vi "Create Dis.vi"(0 "reference in":refnum<class "Stand.lvclass">, 11 "error in (no error)":errorcluster) -> (4 "reference out":refnum<class "Stand.lvclass">, 15 "error out":errorcluster)   [LabVIEW 2019, in "Stand.lvclass"]
uses:
  Stand.lvclass
  C:/Users/ANENKOV_V1/Desktop/src/Proccess_class/Proccess.lvclass
  Stand.lvclass/Stand.ctl
  Proccess_class/Proccess.lvclass/Proccess.ctl
  Proccess_class/TAGs.ctl
  DI_class/DI.lvclass
  Proccess_class/Proccess.lvclass
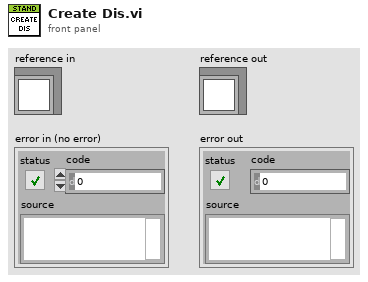
[diagram p1: front panel]
types:
  T1 = typedef "Proccess.lvclass/TAGs.ctl" = cluster{"TAG":string, "PTAG":string, "DESC":string}
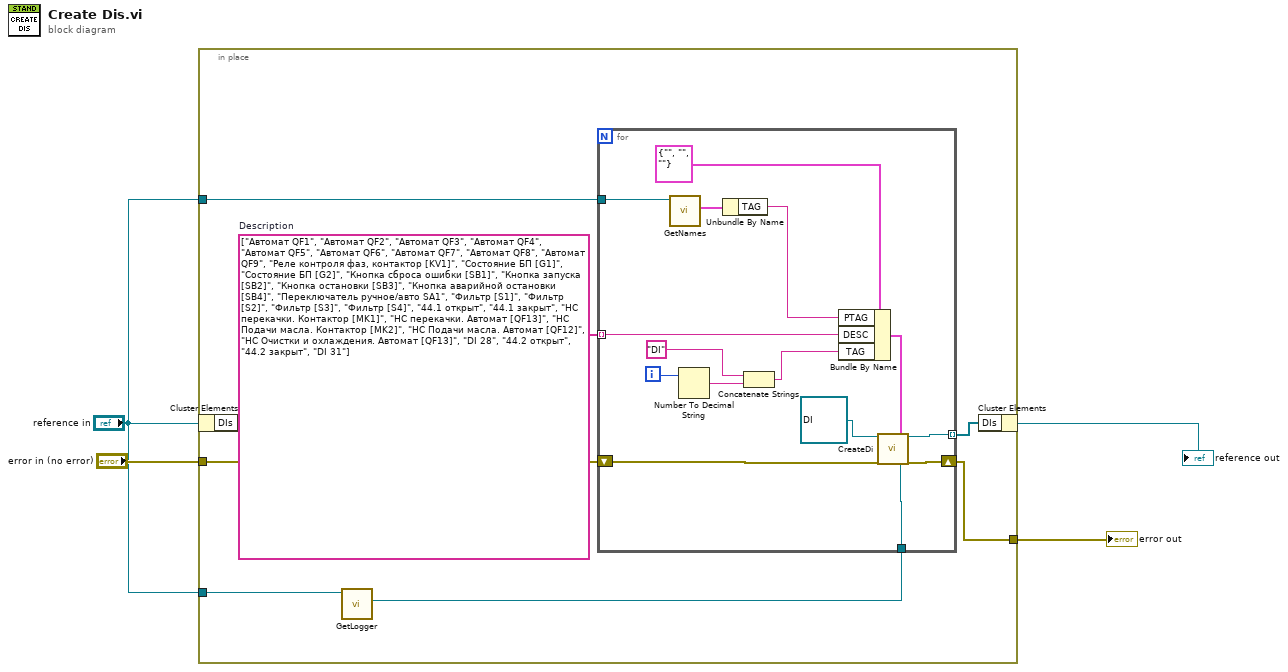
[diagram p0: block diagram]
diagram:
  n1 = in-place {
    in-place-border: "error in (no error)" -> [w11]
    in-place-border: "reference in" -> [w9]
    in-place-border: "reference in" -> [w8]
    in-place-border: [w5] -> w4
    w6 = string[] ["Автомат QF1", "Автомат QF2", "Автомат QF3", "Автомат QF4", "Автомат QF5", "Автомат QF6", "Автомат QF7", "Автомат QF8", "Автомат QF9", "Реле контроля фаз, контактор [KV1]", "Состояние БП [G1]", "Состояние БП [G2]", "Кнопка сброса ошибки [SB1]", "Кнопка запуска [SB2]", "Кнопка остановки [SB3]", "Кнопка аварийной остановки [SB4]", "Переключатель ручное/авто SA1", "Фильтр [S1]", "Фильтр [S2]", "Фильтр [S3]", "Фильтр [S4]", "44.1 открыт", "44.1 закрыт", "НС перекачки. Контактор [MK1]", "НС перекачки. Автомат [QF13]", "НС Подачи масла. Контактор [MK2]", "НС Подачи масла. Автомат [QF12]", "НС Очистки и охлаждения. Автомат [QF13]", "DI 28", "44.2 открыт", "44.2 закрыт", "DI 31"]  # Description
    n2 = in-place-cluster #1("reference in") -> ()  [unwired: 1 out]
    n3 = call "GetLogger.vi"("Proccess in"=w8) -> ("Logger"=w7:refnum<class "Logger.lvclass">)  [unwired: 10 in]
    n4 = for {
      tunnel: [w22] -> w10 mode=indexing
      shift-right: [w21] -> w5
      shift-left: w11 -> [w23]
      tunnel: w6 -> [w17] mode=indexing
      tunnel: w9 -> [w14]
      tunnel: w7 -> [w13]
      i -> [w26]
      n5 = call "GetNames.vi"("Proccess in"=w14) -> ("Tags"=w16:T1)  [unwired: 10 in]
      n6 = Number To Decimal String(number=w26) -> (decimal integer string=w25:string)  [unwired: 1 in]
      n7 = Unbundle By Name(w16) -> ("TAG"=w15:string)
      n8 = Concatenate Strings("DI" ("string"), w25) -> (w18:string)
      n9 = Bundle By Name(cluster=T1 {"TAG"="", "PTAG"="", "DESC"=""} ("Tags"), "PTAG"=w15, "DESC"=w17, "TAG"=w18) -> (w19:T1)
      n10 = call "CreateDi.vi"("Sig_DI_Simple in"=refnum<class "DI.lvclass"> refnum, "error in (no error)"=w23, "Tags"=w19, "Logger"=w13) -> ("Sig_DI_Simple out"=w22:refnum<class "DI.lvclass">, "error out"=w21:errorcluster)  [unwired: 14 in]
    }
    n11 = in-place-cluster #1("DIs"=w10) -> (→"reference out":refnum<class "Stand.lvclass">)
  }
  "error out" <- w4
